vi "parseModuleString.vi"(8 "error in (no error)":errorcluster, 11 "Module in":refnum<class "Module.lvclass">) -> (0 "error out":errorcluster, 3 "Module out":refnum<class "Module.lvclass">)   [LabVIEW 2016, in "Module.lvclass"]
uses:
  Module.lvclass
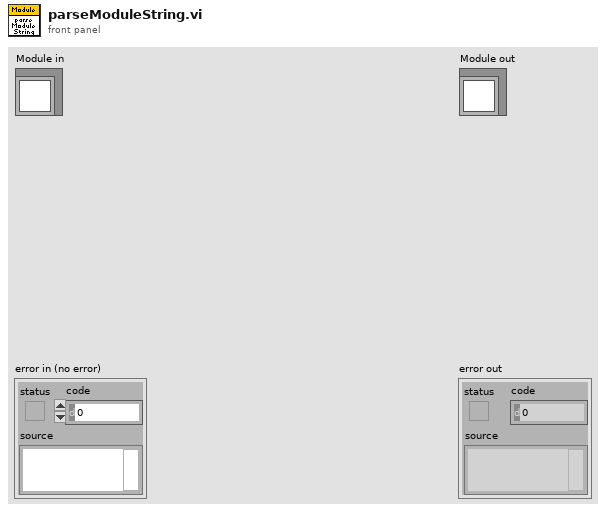
[diagram p1: front panel]
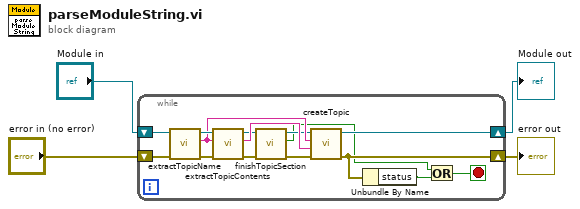
[diagram p0: block diagram]
diagram:
  n1 = while {
    shift-right: [w11] -> w3
    shift-left: "error in (no error)" -> [w13]
    shift-right: [w10] -> w1
    shift-left: "Module in" -> [w17]
    stop <- w18 stop-if-true
    n2 = call "extractTopicName.vi"("error in (no error)"=w13, "Module in"=w17) -> ("error out"=w12:errorcluster, "topicName"=w15:string, "Module out"=w16:refnum<class "Module.lvclass">)  [unwired: 7 in]
    n3 = call "extractTopicContents.vi"("error in (no error)"=w12, "topicName"=w15, "Module in"=w16) -> ("error out"=w7:errorcluster, "topicContentsString"=w14:string, "Module out"=w9:refnum<class "Module.lvclass">)  [unwired: 6 in]
    n4 = call "finishTopicSection.vi"("error in (no error)"=w7, "Module in"=w9) -> ("error out"=w6:errorcluster, "reachedEnd?"=w5:bool, "Module out"=w8:refnum<class "Module.lvclass">)  [unwired: 7 in]
    n5 = call "createTopic.vi"("error in (no error)"=w6, "topicContentsString"=w14, "topicName"=w15, "Module in"=w8) -> ("error out"=w11:errorcluster, "Module out"=w10:refnum<class "Module.lvclass">)  [unwired: 6 in]
    n6 = Unbundle By Name(w11) -> ("status"=w19:bool)
    n7 = Or(x=w5, y=w19) -> (x .or. y?=w18:bool)
  }
  "error out" <- w3
  "Module out" <- w1
